vi "Mask Color.vi"(2 "Current Mask Color":u32(colorbox), 3 "mask data":T1={"image type"=0, "image depth"=24, "image"=array[302784 elements], "mask"=[], "colors"=[], "Rectangle"={"left"=0, "top"=0, "right"=332, "bottom"=304}}, 4 "image data":T1={"image type"=0, "image depth"=24, "image"=array[171063 elements], "mask"=[], "colors"=[], "Rectangle"={"left"=0, "top"=0, "right"=249, "bottom"=229}}) -> (1 "Picture":picture)   [LabVIEW 2010]
doc: "Masking is used when you don't want to draw certain colors of an image onto the picture control. This means that if an image has already been drawn onto the control, then masking out certain colors makes those sections of the new picture appear transparent with the original picture showing through. Multiple colors can be masked by using the combine mask option, and selecting all the colors that you want to mask out.\n\nThis example also shows how the current image in a picture control can be saved to a JPEG or bitmap file."
uses:
  <vilib>/picture/picture.llb/imagedata.ctl
panel:
  # "Click on the color that you want to mask out, and watch the original \npicture become visible. Turn the Combine Masks option 'On' to combine \nall previous masks and mask more than one color at a time."
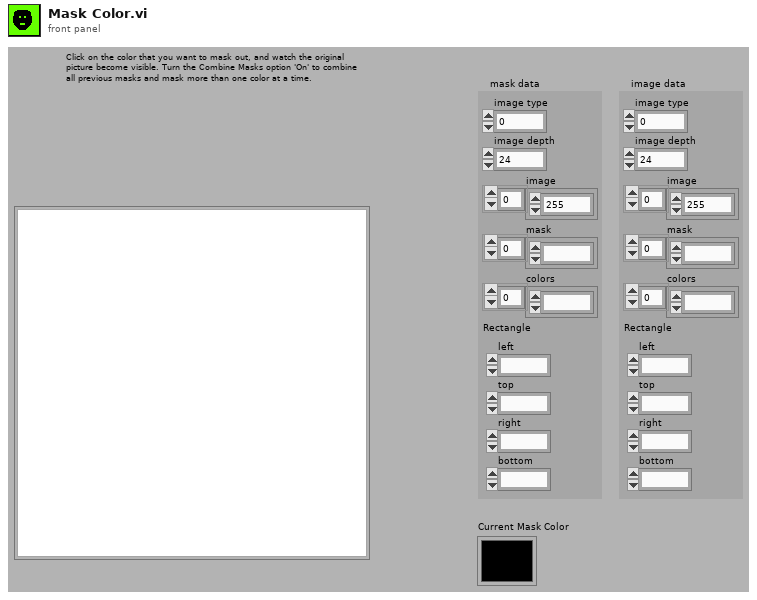
[diagram p1: front panel]
types:
  T1 = typedef "imagedata.ctl" = cluster{"image type":i32, "image depth":i32, "image":u8[], "mask":u8[], "colors":u32[], "Rectangle":cluster{"left":i16, "top":i16, "right":i16, "bottom":i16}}
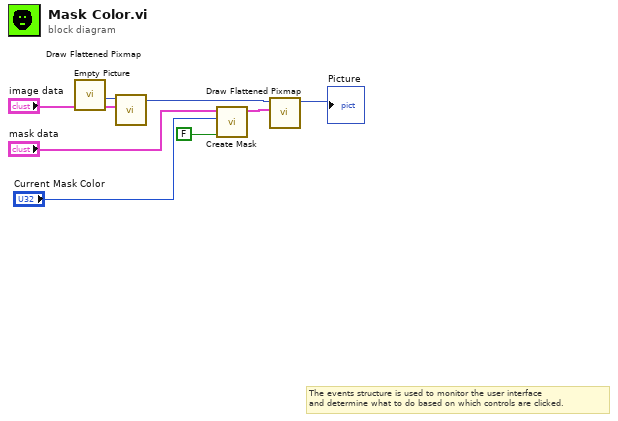
[diagram p0: block diagram]
diagram:
  # "The events structure is used to monitor the user interface \nand determine what to do based on which controls are clicked."
  n1 = call "Empty Picture"() -> ("empty picture"=w8:picture)
  n2 = call <vilib>:"Draw Flattened Pixmap.vi"("image data"="image data", "picture"=w8) -> ("new picture"=w6:picture)  [unwired: 7 in]
  n3 = call <vilib>:"Create Mask.vi"("Combine Masks? (F)"=FALSE, "Mask Color (Black)"="Current Mask Color", "image data"="mask data") -> ("image data"=w3:T1)  [unwired: 8 in]
  n4 = call <vilib>:"Draw Flattened Pixmap.vi"("image data"=w3, "picture"=w6) -> ("new picture"=→"Picture":picture)  [unwired: 7 in]
